vi "ATI InTrap-MALDI Explorer.vi"() -> ()   [LabVIEW 2018]
uses:
  PublicSubVI/Class/FileManager/FM/ctl/_PC_Pub_FM ctrlFileRefnumEnum.ctl
  PublicSubVI/Ctl/RegistyFunc.ctl
  PublicSubVI/Class/FileManager/FM/ctl/_PC_Pub_FM stateMachineEnum.ctl
  PublicSubVI/Class/QMH/QMH.lvclass
  PublicSubVI/Class/DataXML/DataXML.lvclass
  PublicSubVI/Class/Sig2MS/Sig2MS.lvclass
  PublicSubVI/Class/FileManager/FM.lvclass
panel:
  in  "TIC_enable":bool
  in  "Sys.Settings":bool
  in  "MS.RecipeEditor":bool
  in  "MS.Laser":bool
  in  "MS.Turbo":bool
  in  "MS.IonSource":bool
  in  "MS.Pause":bool
  in  "RemainingLoops":i32=-1
  in  "MS.Start":bool
  in  "MS.Config":bool
  in  "warning sign":bool
  in  "eng_mode_str":string
  in  "interface type":enum16{"User", "Engineer"}(ring)
  out "Stop":bool
  in  "Add GroupName":bool
  in  "Auto Index":bool
  in  "Save Config":bool
  in  "Working Folder":path
  in  "MS.AVG":u8=1 min=1 step=1
  in  "MS.Loops":i32=1 min=1 step=1
  in  "Open TempFiles":bool
  in  "Group Name Selection":string(combo)
  out "Last acq. at":timestamp
  in  "File.Save it":bool
  in  "Config Tab":enum32{"D999", "Instrument"}(tab)
  in  "D999_list":i32(listbox)=-1
  out "Instrument_param_table":string[][](table)
  in  "sys_value_list":i32(listbox)=-1
  in  "D999.Config":bool
  out "timeDomainSpec":waveform(sgl)[](graph)
  in  "AVG :":string
  out "massSpec":cluster{dbl[], sgl[]}[](graph)
  out "TIC_wfm":cluster{dbl[], sgl[]}[](graph)
  out "Ionisation":waveform(sgl)[](graph)
  out "Version :":string
  out "Interrupt Signal":bool
  in  "Smooth.edit":bool
  in  "Time domain":bool
  in  "SigProc":bool
  in  "Pressure:":string
  out "# Signal in Queue":u8(slide) scale=0.0..20.0
  out "# signal in NS":u8(slide) scale=0.0..20.0
  in  "Firmware :":string="Open Variable Connection in _PC_RTLoop_ReadCurrentMSEvent.vi->ATI InTrap-MALDI Explorer.vi"
  in  "SysMsg":string="System disconnected"
  out "Network\nstream":bool
  # "TIC"
  # "System"
  # "MSScript"
  # "MS Periphery"
  # "MS Cmd"
  # "Advanced"
  # "File Mgmt."
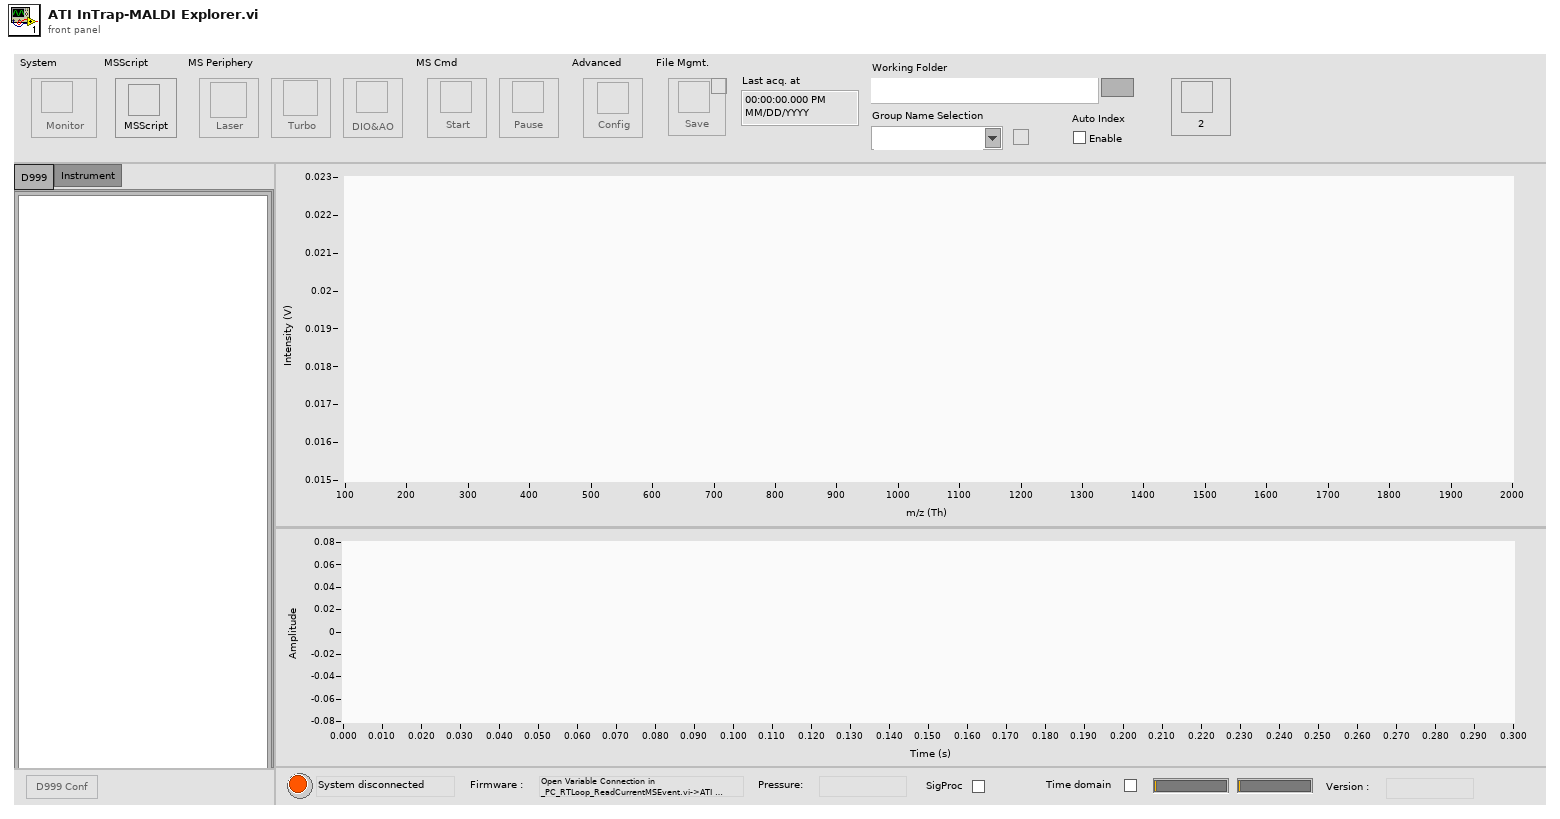
[diagram p1: front panel]
types:
  T1 = cluster{"File.Save it":refnum<vi>, "# Signal in Queue":refnum<vi>, "TIC":refnum<vi>, "Last acq. at":refnum<vi>, "sysValList":refnum<vi>, "signWarning":refnum<vi>, "MS.Pause":refnum<vi>}
  T2 = cluster{"massSpec":refnum<vi>, "timeDomainSpec":refnum<vi>, "Ionisation":refnum<vi>, "Interrupt Signal":refnum<vi>, "AVG":refnum<vi>}
  T3 = enum8{"Enabled", "Disabled", "Disabled and Grayed Out"}
  T4 = cluster{"# signal in NS":refnum<vi>, "# Signal in Queue":refnum<vi>, "MS.Start":refnum<vi>, "MS.Pause":refnum<vi>, "RemainingLoops":refnum<vi>, "Group Name Selection":refnum<vi>, "Add GroupName":refnum<vi>, "Working Folder":refnum<vi>}
  T5 = cluster{"MainVI Ref":refnum<vi>, "D999_list":refnum<vi>, "instr_param_table":refnum<vi>, "sys_value_list":refnum<vi>, "Ionisation":refnum<vi>, "SigProc":refnum<vi>, "Config Tab":refnum<vi>, "MS.RecipeEditor":refnum<vi>, "Open TempFiles":refnum<vi>, "DAQ.Config":refnum<vi>, "Mass spectrum":refnum<vi>, "TIC":refnum<vi>, "fileRefnum":cluster{"folderPath":path, "dataName":string, "fileNameRefnum":refnum<vi>, "workFolderRefnum":refnum<vi>, "openTempFile":refnum<vi>}}
  T6 = cluster{"folderPath":path, "dataName":string, "fileNameRefnum":refnum<vi>, "workFolderRefnum":refnum<vi>, "openTempFile":refnum<vi>}
  T7 = enum16{"init", "loadScript", "newScript", "runScript", "close"}
  T8 = enum16{"None", "Init", "Write", "Read", "PauseRead", "FinishCheck"}
  T9 = cluster{"Method.Path":refnum<data-value>, "MS.Continue":refnum<data-value>, "MS.Loops":refnum<data-value>, "MS.AVG":refnum<data-value>}
  T10 = typedef "_PC_Pub_FM stateMachineEnum.ctl" = enum16{"none", "init", "reset_t0", "openTDMS", "writeTDMS", "closeTDMS", "readTDMS", "getDataItems"}
  T11 = typedef "_PC_Pub_FM ctrlFileRefnumEnum.ctl" = enum16{"init", "checkFileName", "updFileName", "updWorkFolder", "updDataItems", "addNewFileName", "addSerialNum"}
  T12 = typedef "RegistyFunc.ctl" = enum16{"None", "FileAutoSave", "FileNoise", "FileSN", "ExeStatu", "WorkFolderPath", "MethodPath", "AVGItem", "LoopItem", "AutoRun", "BGColor", "LineColor", "LineWidth", "XGrid", "YGrid", "DeviceRefnum"}
  T13 = cluster{"BGColor":u32, "GridX":bool, "GridY":bool, "LineColorArray":u32[], "LineWidthArray":u8[]}
  T14 = typedef "LVPoint32TypeDef.ctl" = cluster{"Horizontal":i32, "Vertical":i32}
  T15 = typedef "LVRowAndColumnTypeDef.ctl" = cluster{"Row":i32, "Column":i32}
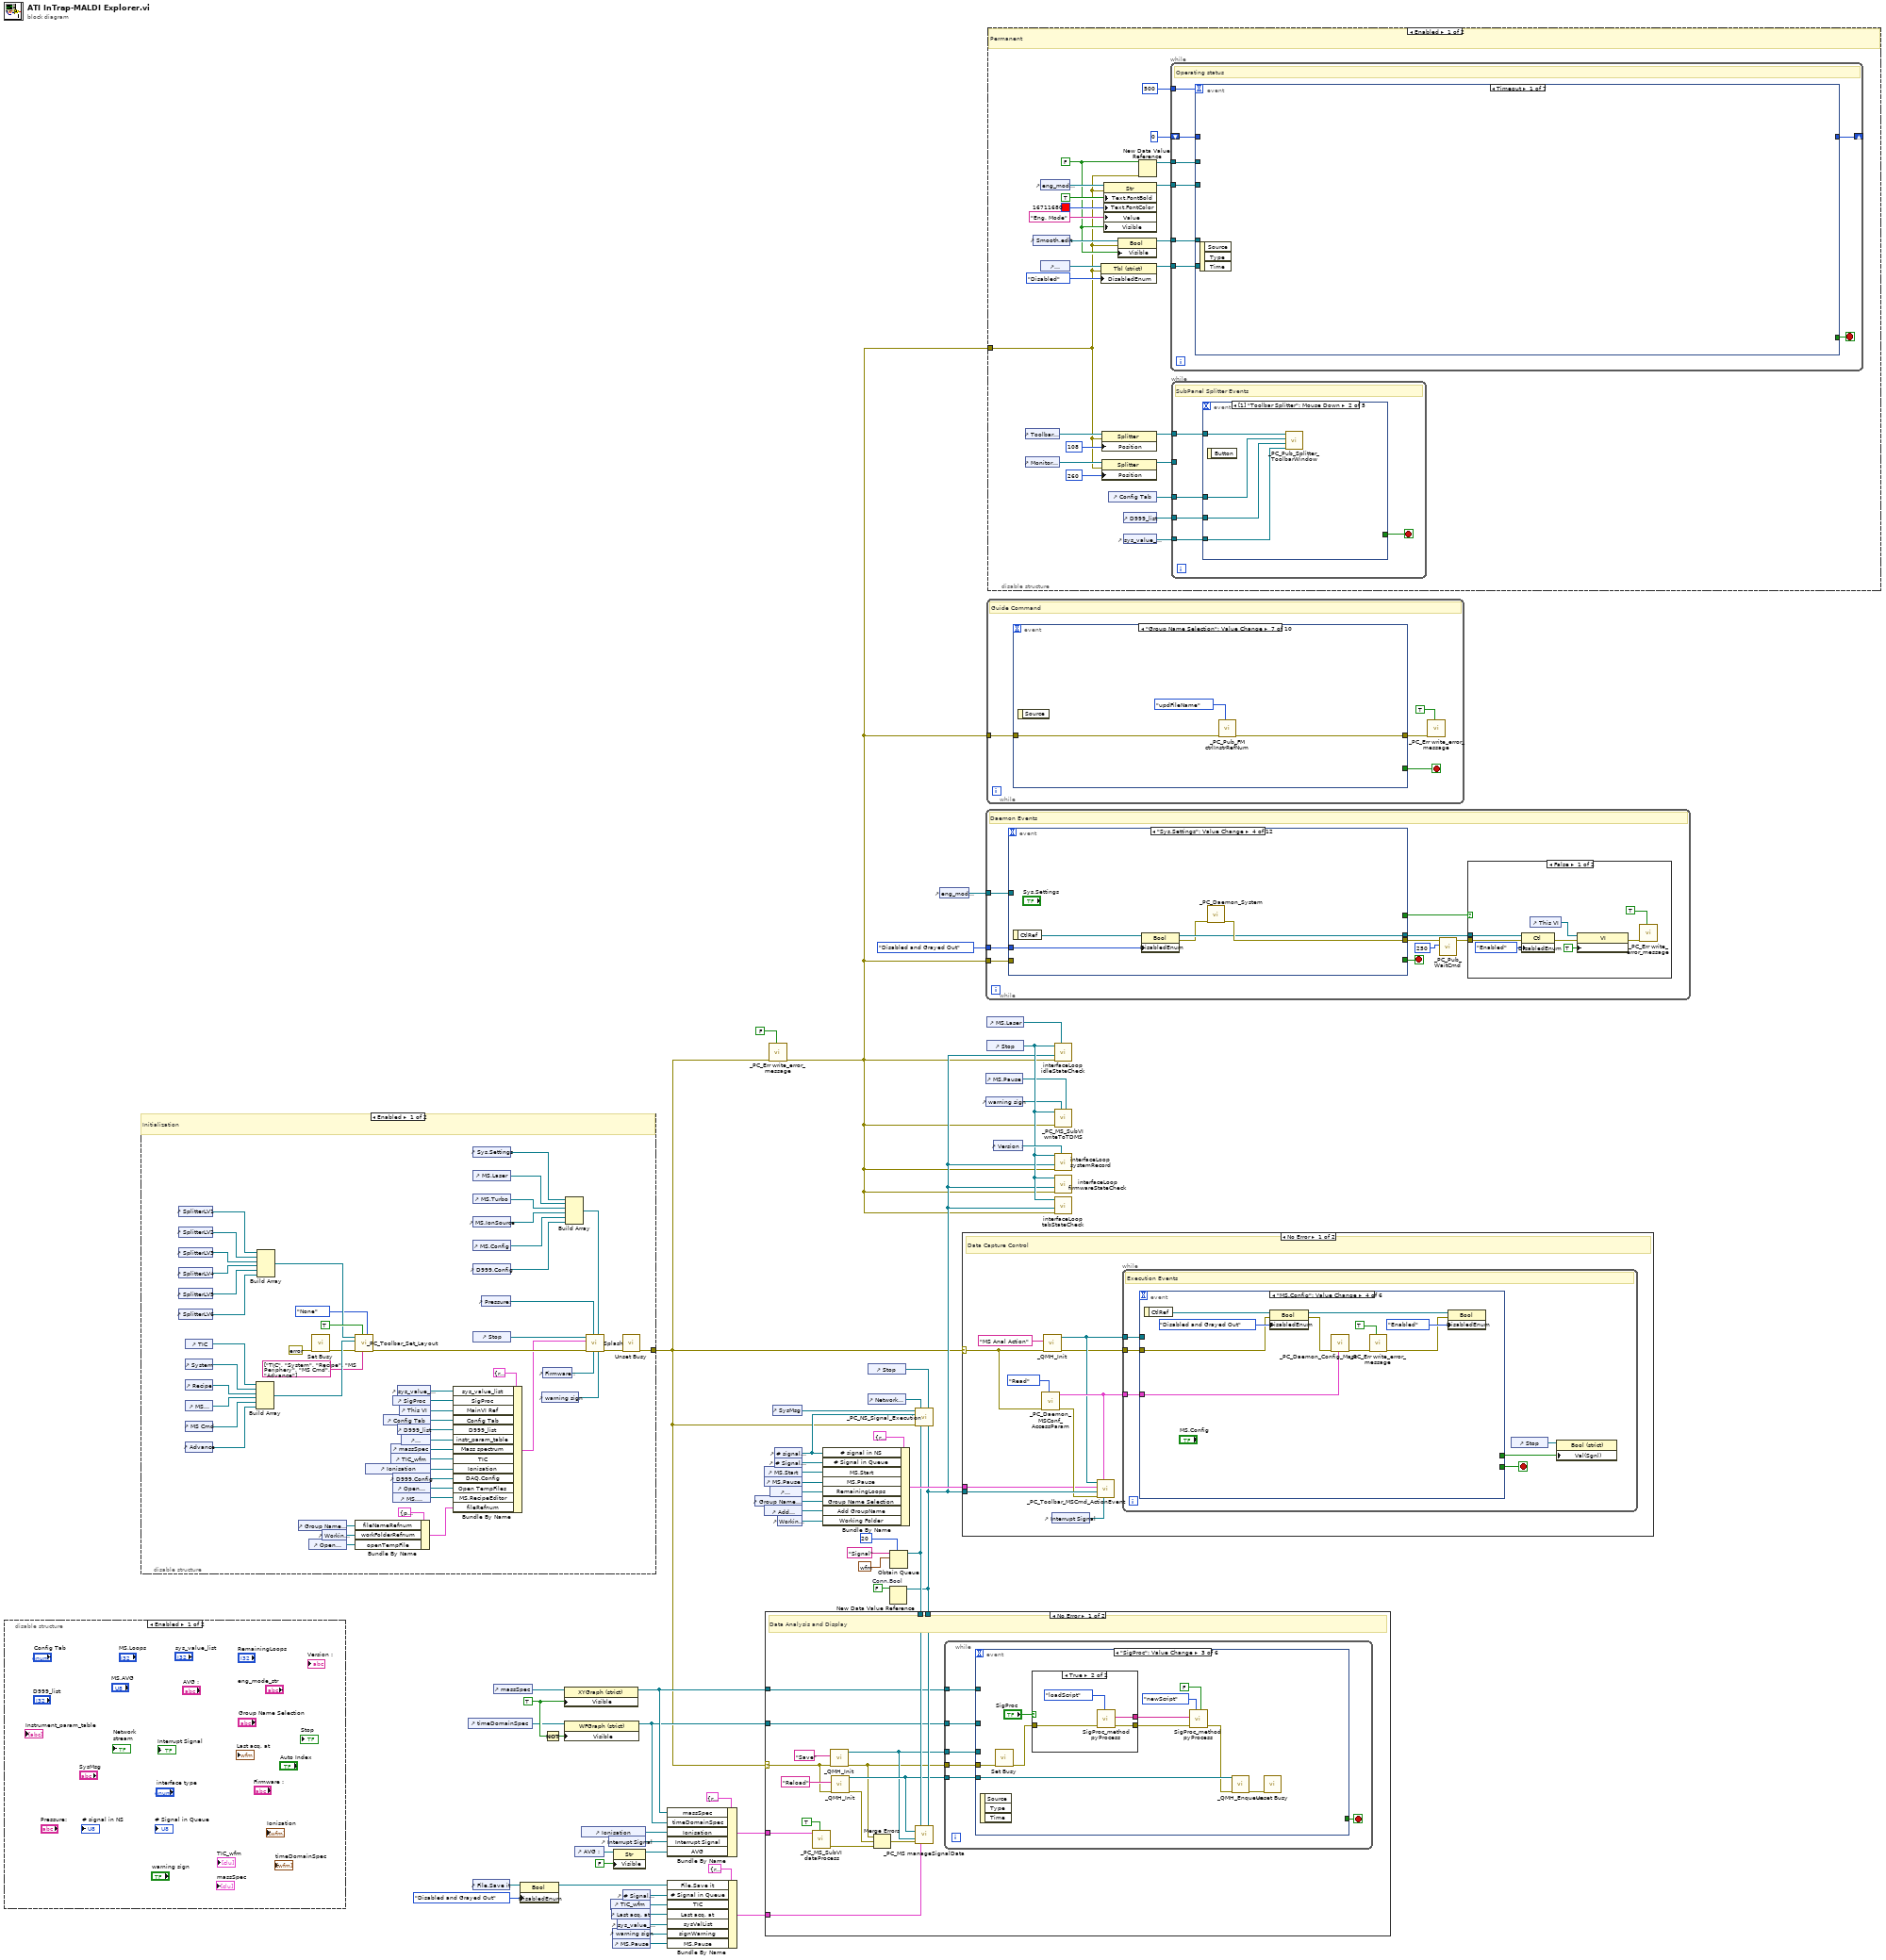
[diagram p0: block diagram]
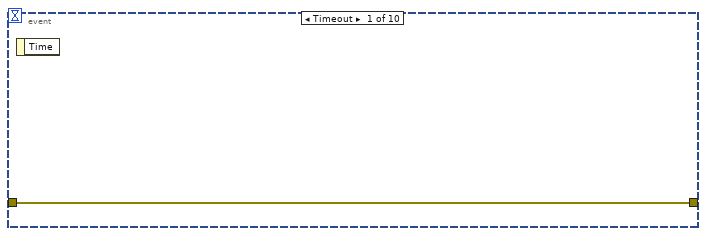
[diagram p2: hidden frame]
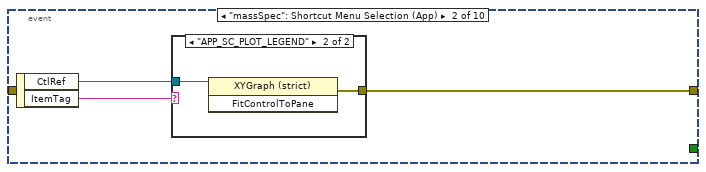
[diagram p3: hidden frame]
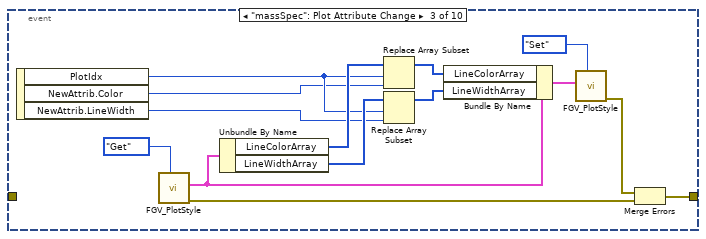
[diagram p5: hidden frame]
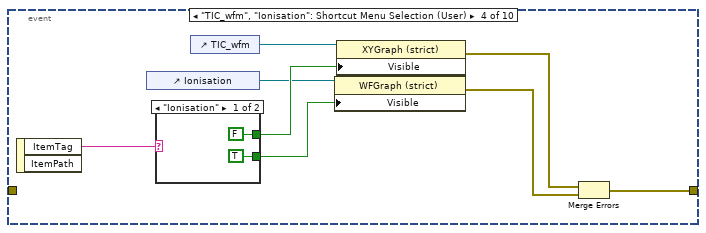
[diagram p6: hidden frame]
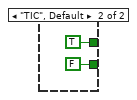
[diagram p7: hidden frame]
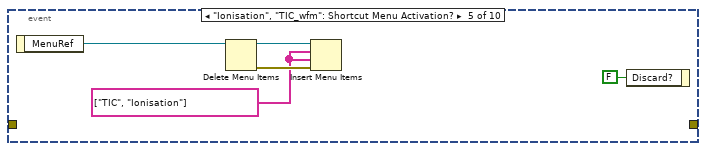
[diagram p8: hidden frame]
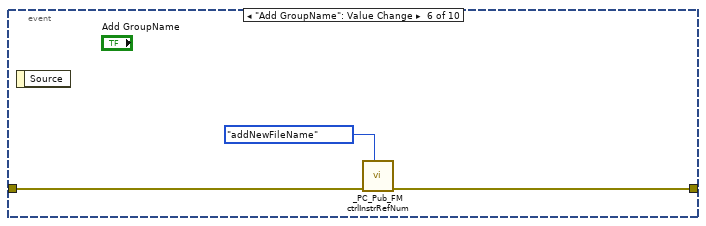
[diagram p9: hidden frame]
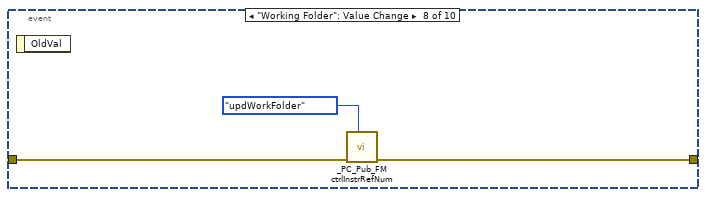
[diagram p10: hidden frame]
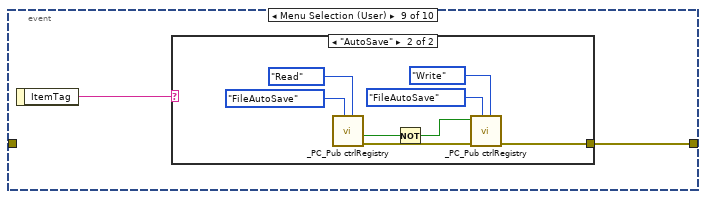
[diagram p11: hidden frame]
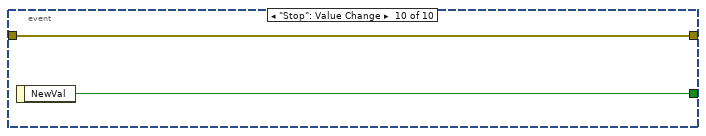
[diagram p13: hidden frame]
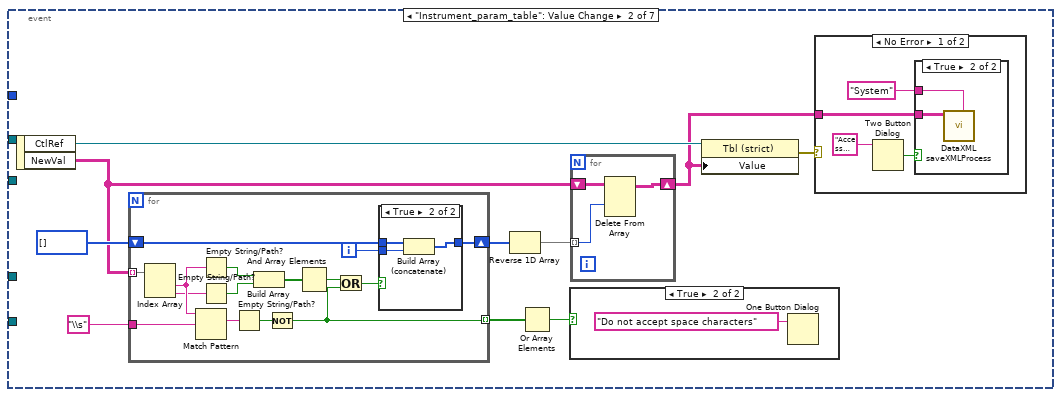
[diagram p14: hidden frame]
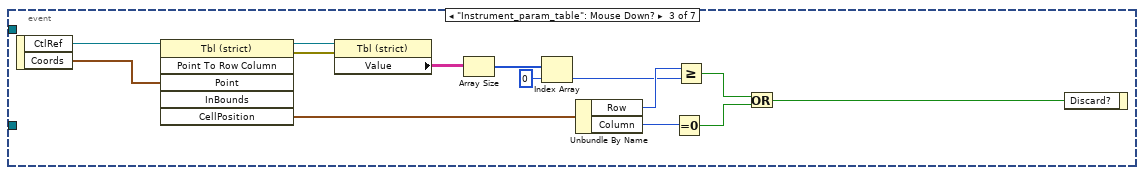
[diagram p19: hidden frame]
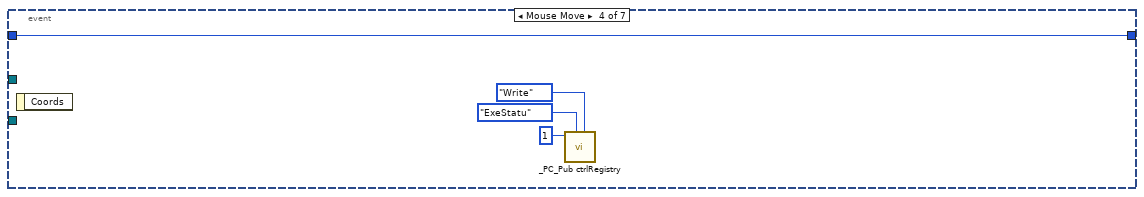
[diagram p20: hidden frame]
diagram:
  w26 = TRUE ("Visible")
  n1 = disable-structure shown="Enabled" {
    frame Enabled {
    }
    frame Disabled {
    }
  }
  n2 = disable-structure shown="Enabled" {
    disable-tunnel: [w105 _] -> w2
    frame Enabled {
      # "Initialization"
      n3 = control-ref of="SplitterLV1"() -> (w99:refnum<vi>)
      n4 = control-ref of="SplitterLV2"() -> (w98:refnum<vi>)
      n5 = control-ref of="SplitterLV3"() -> (w97:refnum<vi>)
      n6 = control-ref of="SplitterLV4"() -> (w96:refnum<vi>)
      n7 = control-ref of="SplitterLV5"() -> (w95:refnum<vi>)
      n8 = control-ref of="SplitterLV6"() -> (w94:refnum<vi>)
      n9 = control-ref of="TIC"() -> (w93:refnum<vi>)
      n10 = control-ref of="System"() -> (w92:refnum<vi>)
      n11 = control-ref of="Recipe"() -> (w91:refnum<vi>)
      n12 = control-ref of="MS Periphery"() -> (w90:refnum<vi>)
      n13 = control-ref of="MS Cmd"() -> (w88:refnum<vi>)
      n14 = control-ref of="Advance"() -> (w89:refnum<vi>)
      n15 = Build Array(w93, w92, w91, w90, w88, w89) -> (w86:refnum<vi>[])
      n16 = Build Array(w99, w98, w97, w96, w95, w94) -> (w84:refnum<vi>[])
      n17 = control-ref of="Group Name Selection"() -> (w82:refnum<vi>)
      n18 = control-ref of="Open TempFiles"() -> (w57:refnum<vi>)
      n19 = call <vilib>:"Set Busy.vi"("error in (no error)"=errorcluster {"status"=FALSE, "code"=0, "source"=""}) -> ("error out"=w81:errorcluster)  [unwired: 9 in, 1 out]
      n20 = control-ref of="Working Folder"() -> (w58:refnum<vi>)
      n21 = call "_PC_Toolbar_Set_Layout.vi"("MachineType"=enum16{"None", "MALDI", "ESI"}."None", "TagArray"=string[] ["TIC", "System", "Recipe", "MS Periphery", "MS Cmd", "Advance"], "Init?(F)"=TRUE, "error in (no error)"=w81, "PanelRef_Array"=w86, "SplitterRef_Array"=w84) -> ("error out"=w69:errorcluster)  [unwired: 5 in]
      n22 = Bundle By Name(cluster=T6 {"folderPath"=path "", "dataName"="", "fileNameRefnum"=refnum, "workFolderRefnum"=refnum, "openTempFile"=refnum} ("fileRefnum"), "fileNameRefnum"=w82, "workFolderRefnum"=w58, "openTempFile"=w57) -> (w56:T6)
      n23 = control-ref of="Ionisation"() -> (w100:refnum<vi>)
      n24 = control-ref of="Config Tab"() -> (w67:refnum<vi>)
      n25 = control-ref of="massSpec"() -> (w102:refnum<vi>)
      n26 = control-ref of="TIC_wfm"() -> (w101:refnum<vi>)
      n27 = control-ref of="SigProc"() -> (w64:refnum<vi>)
      n28 = control-ref of="D999.Config"() -> (w80:refnum<vi>)
      n29 = control-ref of="Open TempFiles"() -> (w79:refnum<vi>)
      n30 = control-ref of="MS.RecipeEditor"() -> (w78:refnum<vi>)
      n31 = control-ref of="sys_value_list"() -> (w63:refnum<vi>)
      n32 = control-ref of="D999_list"() -> (w103:refnum<vi>)
      n33 = control-ref of="This VI"() -> (w77:refnum<vi>)
      n34 = control-ref of="Instrument_param_table"() -> (w65:refnum<vi>)
      n35 = Bundle By Name(cluster=T5 {"MainVI Ref"=refnum, "D999_list"=refnum, "instr_param_table"=refnum, "sys_value_list"=refnum, "Ionisation"=refnum, "SigProc"=refnum, "Config Tab"=refnum, "MS.RecipeEditor"=refnum, "Open TempFiles"=refnum, "DAQ.Config"=refnum, "Mass spectrum"=refnum, "TIC"=refnum, "fileRefnum"={"folderPath"=path "", "dataName"="", "fileNameRefnum"=refnum, "workFolderRefnum"=refnum, "openTempFile"=refnum}} ("Init Ref"), "sys_value_list"=w63, "SigProc"=w64, "MainVI Ref"=w77, "Config Tab"=w67, "D999_list"=w103, "instr_param_table"=w65, "Mass spectrum"=w102, "TIC"=w101, "Ionisation"=w100, "DAQ.Config"=w80, "Open TempFiles"=w79, "MS.RecipeEditor"=w78, "fileRefnum"=w56) -> (w55:T5)
      n36 = control-ref of="Sys.Settings"() -> (w75:refnum<vi>)
      n37 = control-ref of="MS.Laser"() -> (w74:refnum<vi>)
      n38 = control-ref of="MS.Turbo"() -> (w73:refnum<vi>)
      n39 = control-ref of="MS.IonSource"() -> (w72:refnum<vi>)
      n40 = control-ref of="MS.Config"() -> (w66:refnum<vi>)
      n41 = control-ref of="D999.Config"() -> (w71:refnum<vi>)
      n42 = control-ref of="Stop"() -> (w68:refnum<vi>)
      n43 = control-ref of="Pressure:"() -> (w70:refnum<vi>)
      n44 = control-ref of="warning sign"() -> (w61:refnum<vi>)
      n45 = control-ref of="Firmware :"() -> (w62:refnum<vi>)
      n46 = Build Array(w75, w74, w73, w72, w66, w71) -> (w104:refnum<vi>[])
      n47 = call "Splash.vi"("warning sign"=w61, "Cluster control array"=w104, "Firmware :"=w62, "Pressure:"=w70, "error in (no error)"=w69, "Init Ref"=w55, "Stop"=w68) -> ("error out"=w60:errorcluster)  [unwired: 4 in]
      n48 = call <vilib>:"Unset Busy.vi"("error in (no error)"=w60) -> ("error out"=w105:errorcluster)  [unwired: 10 in]
    }
    frame Disabled {
    }
  }
  n49 = control-ref of="timeDomainSpec"() -> (w23:refnum<vi>)
  n50 = control-ref of="File.Save it"() -> (w49:refnum<vi>)
  n51 = control-ref of="massSpec"() -> (w24:refnum<vi>)
  n52 = property class="Bool"(reference=w49, "DisabledEnum"=T3."Disabled and Grayed Out" ("Disabled")) -> (reference out=w48:refnum<vi>)  [unwired: 1 in, 1 out]
  n53 = Not(x=w26) -> (.not. x?=w25:bool)
  n54 = property class="XYGraph (strict)"(reference=w24, "Visible"=w26) -> (reference out=w22:refnum<vi>)  [unwired: 1 in, 1 out]
  n55 = property class="WFGraph (strict)"(reference=w23, "Visible"=w25) -> (reference out=w19:refnum<vi>)  [unwired: 1 in, 1 out]
  n56 = control-ref of="AVG :"() -> (w20:refnum<vi>)
  n57 = control-ref of="Ionisation"() -> (w21:refnum<vi>)
  n58 = control-ref of="Interrupt Signal"() -> (w17:refnum<vi>)
  n59 = control-ref of="TIC_wfm"() -> (w51:refnum<vi>)
  n60 = control-ref of="Last acq. at"() -> (w53:refnum<vi>)
  n61 = control-ref of="warning sign"() -> (w14:refnum<vi>)
  n62 = control-ref of="MS.Pause"() -> (w13:refnum<vi>)
  n63 = property class="Str"(reference=w20, "Visible"=FALSE) -> (reference out=w16:refnum<vi>)  [unwired: 1 in, 1 out]
  n64 = control-ref of="sys_value_list"() -> (w15:refnum<vi>)
  n65 = control-ref of="# Signal in Queue"() -> (w52:refnum<vi>)
  n66 = Bundle By Name(cluster=T1 {"File.Save it"=refnum, "# Signal in Queue"=refnum, "TIC"=refnum, "Last acq. at"=refnum, "sysValList"=refnum, "signWarning"=refnum, "MS.Pause"=refnum}, "File.Save it"=w48, "# Signal in Queue"=w52, "TIC"=w51, "Last acq. at"=w53, "sysValList"=w15, "signWarning"=w14, "MS.Pause"=w13) -> (w42:T1)
  n67 = Bundle By Name(cluster=T2 {"massSpec"=refnum, "timeDomainSpec"=refnum, "Ionisation"=refnum, "Interrupt Signal"=refnum, "AVG"=refnum} ("Reference"), "massSpec"=w22, "timeDomainSpec"=w19, "Ionisation"=w21, "Interrupt Signal"=w17, "AVG"=w16) -> (w40:T2)
  n68 = control-ref of="Group Name Selection"() -> (w6:refnum<vi>)
  n69 = control-ref of="MS.Start"() -> (w31:refnum<vi>)
  n70 = control-ref of="MS.Pause"() -> (w27:refnum<vi>)
  n71 = control-ref of="Add GroupName"() -> (w5:refnum<vi>)
  n72 = call "_PC_Err write_error_message.vi"("show msg( T )"=FALSE, "error in"=w2) -> ("error out"=w1:errorcluster)  [unwired: 9 in]
  n73 = control-ref of="RemainingLoops"() -> (w33:refnum<vi>)
  n74 = control-ref of="SysMsg"() -> (w44:refnum<vi>)
  n75 = control-ref of="# signal in NS"() -> (w43:refnum<vi>)
  n76 = control-ref of="# Signal in Queue"() -> (w46:refnum<vi>)
  n77 = control-ref of="Working Folder"() -> (w4:refnum<vi>)
  n78 = Bundle By Name(cluster=T4 {"# signal in NS"=refnum, "# Signal in Queue"=refnum, "MS.Start"=refnum, "MS.Pause"=refnum, "RemainingLoops"=refnum, "Group Name Selection"=refnum, "Add GroupName"=refnum, "Working Folder"=refnum} ("Cluster"), "# signal in NS"=w43, "# Signal in Queue"=w46, "MS.Start"=w31, "MS.Pause"=w27, "RemainingLoops"=w33, "Group Name Selection"=w6, "Add GroupName"=w5, "Working Folder"=w4) -> (w45:T4)
  n79 = control-ref of="Stop"() -> (w32:refnum<vi>)
  n80 = control-ref of="Network\nstream"() -> (w47:refnum<vi>)
  n81 = New Data Value Reference "Conn.Bool"(data value=FALSE) -> (data value reference=w9:refnum<data-value>)  [unwired: 1 in, 1 out]
  n82 = Obtain Queue(max queue size (-1, unlimited)=20, name (unnamed)="Signal", element data type=waveform(sgl) {"t0"=timestamp(0 s since 1904-01-01), "dt"=1.0, "Y"=[]} ("element")) -> (queue out=w35:refnum<queue>)  [unwired: 2 in, 2 out]
  n83 = case shown="No Error" w2 {
    selector: w2 -> [w116 _]
    tunnel: w35 -> [w121 _]
    tunnel: w9 -> [w120 _]
    tunnel: w42 -> [w115 _]
    tunnel: w40 -> [w113 _]
    tunnel: w22 -> [w108 _]
    tunnel: w19 -> [w107 _]
    frame No Error {
      # "Data Analysis and Display"
      n84 = call "_PC_MS_SubVI dataProcess.vi"("Init?(F)"=TRUE, "Reference"=w113) -> ("error out"=w110:errorcluster)  [unwired: 8 in, 1 out]
      n85 = call "_QMH_Init.vi"("error in (no error)"=w116, "name (unnamed)"="Save") -> ("error out"=w112:errorcluster, "QMH out"=w114:refnum<class "QMH.lvclass">)  [unwired: 8 in]
      n86 = call "_QMH_Init.vi"("error in (no error)"=w116, "name (unnamed)"="Reload") -> ("error out"=w111:errorcluster, "QMH out"=w117:refnum<class "QMH.lvclass">)  [unwired: 8 in]
      n87 = Merge Errors(w112, w111, w110) -> (w109:errorcluster)
      n88 = call "_PC_MS manageSignalData.vi"("Sig Queue"=w121, "Conn_Bool"=w120, "Reload_QMH"=w117, "Save_QMH"=w114, "error in (no error)"=w109, "exeObjRefnum"=w115) -> ()  [unwired: 10 in]
      n89 = while {
        tunnel: w117 -> [w127]
        tunnel: w114 -> [w126]
        tunnel: w112 -> [w125]
        tunnel: w108 -> [w123]
        tunnel: w107 -> [w122]
        stop <- w124 stop-if-true
        n90 = event shown="[2] \"SigProc\": Value Change" {
          selector: _ -> [_ _ _ _ _ _]
          dyn-events: _ -> [_ _ _ _ _ _]
          timeout: _ -> [_ _ _ _ _ _]
          tunnel: w127 -> [_ w135 w147 _ w162 _]
          tunnel: w126 -> [_ _ _ w158 _ _]
          tunnel: w125 -> [_ _ w145 w157 w161 _]
          tunnel: [_ _ _ _ _ w163] -> w124
          tunnel: w123 -> [_ w134 _ _ _ _]
          tunnel: w122 -> [_ w133 _ _ _ _]
          event Timeout {
            n91 = event-data() -> ()  [unwired: 1 in, 3 out]
          }
          event "Time domain": Value Change {
            n92 = event-data() -> ()  [unwired: 1 in, 3 out]
            n93 = Not(x="Time domain") -> (.not. x?=w132:bool)
            n94 = property class="WFGraph (strict)"(reference=w133, "Visible"="Time domain") -> (reference out=w129:refnum<vi>)  [unwired: 1 in, 1 out]
            n95 = property class="XYGraph (strict)"(reference=w134, "Visible"=w132) -> (reference out=w130:refnum<vi>)  [unwired: 1 in, 1 out]
            n96 = case shown="False" "Time domain" {
              tunnel: w130 -> [w138 _]
              tunnel: w129 -> [_ w141]
              tunnel: [w136 w139] -> w128
              frame False {
                n97 = property class="XYGraph (strict)"(reference=w138, "Value"=cluster{dbl[], sgl[]}[] []) -> (error out=w136:errorcluster)  [unwired: 1 in, 1 out]
              }
              frame True {
                n98 = property class="WFGraph (strict)"(reference=w141, "Value"=waveform(dbl)[] []) -> (error out=w139:errorcluster)  [unwired: 1 in, 1 out]
              }
            }
            n99 = call "_QMH_Enqueue.vi"("error in (no error)"=w128, "QMH in"=w135) -> ()  [unwired: 8 in, 2 out]
          }
          event "SigProc": Value Change {
            n100 = event-data() -> ()  [unwired: 1 in, 3 out]
            n101 = call <vilib>:"Set Busy.vi"("error in (no error)"=w145) -> ("error out"=w144:errorcluster)  [unwired: 9 in, 1 out]
            n102 = case shown="True" "SigProc" {
              tunnel: [_ w155] -> w149
              tunnel: [w152 w154] -> w148
              tunnel: w144 -> [w152 w153]
              frame False {
              }
              frame True {
                n103 = call "SigProc_method pyProcess.vi"("func"=T7."loadScript", "error in (no error)"=w153) -> ("error out"=w154:errorcluster, "pyCode"=w155:string)  [unwired: 6 in, 2 out]
              }
            }
            n104 = call "SigProc_method pyProcess.vi"("replace?(T)"=FALSE, "func"=T7."newScript", "error in (no error)"=w148, "newScriptCode"=w149) -> ("error out"=w146:errorcluster)  [unwired: 4 in, 3 out]
            n105 = call "_QMH_Enqueue.vi"("error in (no error)"=w146, "QMH in"=w147) -> ("error out"=w143:errorcluster)  [unwired: 8 in, 1 out]
            n106 = call <vilib>:"Unset Busy.vi"("error in (no error)"=w143) -> ()  [unwired: 10 in, 1 out]
          }
          event "File.Save it": Value Change {
            n107 = event-data() -> ()  [unwired: 1 in, 1 out]
            n108 = call "_QMH_Enqueue.vi"("error in (no error)"=w157, "Msg"="Save", "QMH in"=w158) -> ()  [unwired: 7 in, 2 out]
          }
          event "Smooth.edit": Value Change {
            n109 = event-data() -> ()  [unwired: 1 in, 1 out]
            n110 = call "Sig2MS dialogPyScript.vi"("error in (no error)"=w161) -> ("error out"=w160:errorcluster)  [unwired: 10 in]
            n111 = call "_QMH_Enqueue.vi"("error in (no error)"=w160, "QMH in"=w162) -> ()  [unwired: 8 in, 2 out]
          }
          event "Stop": Value Change {
            n112 = event-data() -> ("NewVal"=w163:bool)  [unwired: 1 in]
          }
        }
      }
    }
    frame Error {
    }
  }
  n113 = call "_PC_NS_Signal_Execution.vi"("SysMsg"=w44, "Network\nstream"=w47, "Stop"=w32, "# signal in NS"=w43, "error in (no error)"=w2, "Sig Queue"=w35, "Conn_Bool"=w9) -> ()  [unwired: 9 in]
  n114 = control-ref of="eng_mode_str"() -> (w30:refnum<vi>)
  n115 = case shown="No Error" w2 {
    selector: w2 -> [w166 w240]
    tunnel: w9 -> [w172 _]
    tunnel: w45 -> [w164 _]
    frame No Error {
      # "Data Capture Control"
      n116 = call "_PC_Daemon_MSConf_AccessParam.vi"("Function"=enum16{"Write", "Read"}."Read", "error in (no error)"=w166) -> ("error out"=w168:errorcluster, "exe param memory"=w169:T9)  [unwired: 8 in]
      n117 = call "_QMH_Init.vi"("error in (no error)"=w166, "name (unnamed)"="MS Anal Action") -> ("error out"=w165:errorcluster, "QMH out"=w167:refnum<class "QMH.lvclass">)  [unwired: 8 in]
      n118 = control-ref of="Interrupt Signal"() -> (w171:refnum<vi>)
      n119 = call "_PC_Toolbar_MSCmd_ActionEvent.vi"("Interrupt Signal"=w171, "exe param memory"=w169, "error in (no error)"=w168, "Conn_Bool"=w172, "Cluster"=w164, "QMH In"=w167) -> ()  [unwired: 6 in]
      n120 = while {
        tunnel: w167 -> [w179]
        tunnel: w165 -> [w178]
        tunnel: w169 -> [w177]
        stop <- w174 stop-if-true
        # "Execution Events"
        n121 = event shown="[3] \"MS.Config\": Value Change" {
          selector: _ -> [_ _ _ _ _ _]
          dyn-events: _ -> [_ _ _ _ _ _]
          timeout: _ -> [_ _ _ _ _ _]
          tunnel: w179 -> [_ w195 w209 _ w222 _]
          tunnel: w178 -> [_ w189 w206 w215 w221 _]
          tunnel: w177 -> [_ w192 _ w220 w225 _]
          tunnel: [_ _ _ _ _ TRUE ("stop")] -> w174
          tunnel: [_ _ _ _ TRUE _] -> w175
          event Timeout {
            n122 = event-data() -> ()  [unwired: 1 in, 1 out]
          }
          event "MS.Start": Value Change {
            n123 = event-data() -> ()  [unwired: 1 in, 1 out]
            n124 = Unbundle By Name(w192) -> ("MS.Continue"=w191:refnum<data-value>)
            n125 = call <vilib>:"Set Busy.vi"("error in (no error)"=w189) -> ("error out"=w188:errorcluster)  [unwired: 9 in, 1 out]
            n126 = control-ref of="Ionisation"() -> (w183:refnum<vi>)
            n127 = in-place {
              in-place-border: [w204] -> w199
              in-place-border: w188 -> [_]
              n128 = in-place-dvr #1(w191) -> (w204:bool)  [unwired: 1 out]
              n129 = in-place-dvr #1(w204) -> (w190:errorcluster)  [unwired: 1 out]
            }
            n130 = control-ref of="massSpec"() -> (w194:refnum<vi>)
            n131 = control-ref of="TIC_wfm"() -> (w193:refnum<vi>)
            n132 = control-ref of="Auto Index"() -> (w184:refnum<vi>)
            n133 = Select(t="StartInf" ("Msg"), s=w199, f="Start" ("Msg")) -> (s? t:f=w196:string)
            n134 = call "_PC_MS_SubVI exeInit.vi"("Auto Index"=w184, "error in (no error)"=w190, "Ionisation Ref"=w183, "TIC Ref"=w193, "Mass Spetrum Ref"=w194) -> ("error out"=w182:errorcluster)  [unwired: 6 in]
            n135 = case shown="No Error" w182 {
              selector: w182 -> [w201 _]
              tunnel: w196 -> [w203 _]
              tunnel: w195 -> [w202 _]
              tunnel: [w200 _] -> w187
              frame No Error {
                n136 = call "_QMH_Enqueue.vi"("error in (no error)"=w201, "Msg"=w203, "QMH in"=w202) -> ("error out"=w200:errorcluster)  [unwired: 7 in, 1 out]
              }
              frame Error {
              }
            }
            n137 = call <vilib>:"Clear Errors.vi"("error in (no error)"=w182) -> ("error out"=w181:errorcluster)  [unwired: 5 in, 1 out]
            n138 = call "_PC_Pub_FM ctrlTempStateMachine.vi"("function"=T8."Init", "error in (no error)"=w181) -> ()  [unwired: 7 in, 3 out]
            n139 = call "_PC_Pub_WaitCmd.vi"("milliseconds to wait"=u32 200, "error in (no error)"=w187) -> ("error out"=w186:errorcluster)  [unwired: 9 in]
            n140 = call <vilib>:"Unset Busy.vi"("error in (no error)"=w186) -> ()  [unwired: 10 in, 1 out]
          }
          event "MS.Pause": Value Change {
            n141 = event-data() -> ("CtlRef"=w208:refnum<vi>)  [unwired: 1 in]
            n142 = property class="Bool (strict)"(reference=w208, error in=w206, "DisabledEnum"=T3."Disabled and Grayed Out" ("Disabled")) -> (error out=w205:errorcluster)  [unwired: 1 out]
            n143 = call "_QMH_Enqueue.vi"("error in (no error)"=w205, "Msg"="Pause", "QMH in"=w209) -> ()  [unwired: 7 in, 2 out]
          }
          event "MS.Config": Value Change {
            n144 = event-data() -> ("CtlRef"=w216:refnum<vi>)  [unwired: 1 in]
            n145 = property class="Bool"(reference=w216, error in=w215, "DisabledEnum"=T3."Disabled and Grayed Out" ("Disabled")) -> (reference out=w213:refnum<vi>, error out=w214:errorcluster)
            n146 = call "_PC_Daemon_Config_Mass.vi"("exe param memory"=w220, "error in (no error)"=w214) -> ("error out"=w219:errorcluster)  [unwired: 9 in]
            n147 = call "_PC_Err write_error_message.vi"("show msg( T )"=TRUE, "error in"=w219) -> ("error out"=w211:errorcluster)  [unwired: 9 in]
            n148 = property class="Bool"(reference=w213, error in=w211, "DisabledEnum"=T3."Enabled" ("Disabled")) -> ()  [unwired: 2 out]
          }
          event Panel Close? {
            n149 = event-data() -> ()  [unwired: 1 in, 1 out]
            n150 = Unbundle By Name(w225) -> ("Method.Path"=w231:refnum<data-value>, "MS.Continue"=w228:refnum<data-value>, "MS.Loops"=w229:refnum<data-value>, "MS.AVG"=w230:refnum<data-value>)
            n151 = Delete Data Value Reference(data value reference=w230) -> (error out=w232:errorcluster)  [unwired: 1 in, 1 out]
            n152 = Delete Data Value Reference(data value reference=w229, error in=w232) -> (error out=w233:errorcluster)  [unwired: 1 out]
            n153 = Delete Data Value Reference(data value reference=w228, error in=w233) -> (error out=w234:errorcluster)  [unwired: 1 out]
            n154 = call "_QMH_Enqueue.vi"("error in (no error)"=w221, "Msg"="Close", "QMH in"=w222) -> ("error out"=w235:errorcluster)  [unwired: 7 in, 1 out]
            n155 = Delete Data Value Reference(data value reference=w231, error in=w234) -> (error out=w236:errorcluster)  [unwired: 1 out]
            n156 = Merge Errors(w235, w236) -> (w223:errorcluster)
            n157 = call "_PC_Err write_error_message.vi"("show msg( T )"=FALSE, "error in"=w223) -> ()  [unwired: 9 in, 1 out]
            n158 = event-data() -> ()  [unwired: 2 in, 1 out]
          }
          event Panel Close {
            n159 = event-data() -> ()  [unwired: 1 in, 1 out]
          }
        }
        n160 = control-ref of="Stop"() -> (w176:refnum<vi>)
        n161 = property class="Bool (strict)"(reference=w176, "Val(Sgnl)"=w175) -> ()  [unwired: 1 in, 2 out]
      }
    }
    frame Error {
      n162 = call "_PC_Err write_error_message.vi"("show msg( T )"=FALSE, "error in"=w240) -> ("error out"=w238:errorcluster)  [unwired: 9 in]
      n163 = flat-sequence {
        tunnel: w238 -> [_]
        frame #0 {
          n164 = control-ref of="This VI"() -> (w241:refnum<vi>)
          n165 = invoke class="VI" method="FP.Close"(reference=w241) -> ()  [unwired: 2 in, 3 out]
        }
      }
    }
  }
  n166 = while {
    tunnel: w1 -> [w243]
    tunnel: w30 -> [w244]
    tunnel: T3."Disabled and Grayed Out" ("Disabled") -> [w242]
    stop <- w249 stop-if-true
    # "Daemon Events"
    n167 = event shown="[3] \"Sys.Settings\": Value Change" {
      selector: _ -> [_ _ _ _ _ _ _ _ _ _ _ _]
      dyn-events: _ -> [_ _ _ _ _ _ _ _ _ _ _ _]
      timeout: _ -> [_ _ _ _ _ _ _ _ _ _ _ _]
      tunnel: [_ w260 w266 w272 w280 w283 w289 w297 w300 w306 w330 _] -> w250
      tunnel: [_ w263 w270 w275 w277 w287 w293 w299 w304 w310 w317 _] -> w245
      tunnel: [_ _ _ _ _ _ _ _ _ _ _ w334] -> w249
      tunnel: [_ _ _ _ _ _ _ _ _ _ _ TRUE ("NewVal")] -> w246
      tunnel: w244 -> [_ _ _ _ w276 w288 w294 _ w305 _ _ _]
      tunnel: w243 -> [_ _ _ _ _ _ _ _ _ _ _ _]
      tunnel: w242 -> [_ w261 w268 w273 w281 w285 w291 w296 w302 w308 w331 _]
      event Timeout {
        n168 = event-data() -> ()  [unwired: 1 in, 1 out]
      }
      event "TIC_enable": Value Change {
        n169 = event-data() -> ("CtlRef"=w262:refnum<vi>)  [unwired: 1 in]
        n170 = property class="Bool"(reference=w262, "DisabledEnum"=w261) -> (reference out=w260:refnum<vi>, error out=w259:errorcluster)  [unwired: 1 in]
        n171 = disable-structure shown="Disabled" {
          disable-tunnel: [w265 _] -> w263
          disable-tunnel: w259 -> [w264 _]
          frame Disabled {
            n172 = call "_PC_Daemon_Chromatogram.vi"(8:w264) -> ("error out"=w265:errorcluster)  [unwired: 10 in]
          }
          frame Enabled {
          }
        }
      }
      event "Save Config": Value Change {
        n173 = event-data() -> ("CtlRef"=w269:refnum<vi>)  [unwired: 1 in]
        n174 = property class="Bool"(reference=w269, "DisabledEnum"=w268) -> (reference out=w266:refnum<vi>, error out=w267:errorcluster)  [unwired: 1 in]
        n175 = call "_PC_Daemon_Config_SaveData.vi"("error in (no error)"=w267) -> ("error out"=w270:errorcluster)  [unwired: 10 in]
      }
      event "Sys.Settings": Value Change {
        n176 = event-data() -> ("CtlRef"=w274:refnum<vi>)  [unwired: 1 in]
        n177 = property class="Bool"(reference=w274, "DisabledEnum"=w273) -> (reference out=w272:refnum<vi>, error out=w271:errorcluster)  [unwired: 1 in]
        n178 = call "_PC_Daemon_System.vi"("error in (no error)"=w271) -> ("error out"=w275:errorcluster)  [unwired: 9 in, 1 out]
      }
      event "MS.RecipeEditor": Value Change {
        n179 = event-data() -> ("CtlRef"=w282:refnum<vi>)  [unwired: 1 in]
        n180 = property class="Bool"(reference=w282, "DisabledEnum"=w281) -> (reference out=w280:refnum<vi>, error out=w278:errorcluster)  [unwired: 1 in]
        n181 = control-ref of="Network\nstream"() -> (w279:refnum<vi>)
        n182 = call "_PC_Daemon_RecipeEditor.vi"("eng_mode_str"=w276, "error in (no error)"=w278, "Network\nstream"=w279) -> ("error out"=w277:errorcluster)  [unwired: 8 in]
      }
      event "MS.Laser": Value Change {
        n183 = event-data() -> ("CtlRef"=w286:refnum<vi>)  [unwired: 1 in]
        n184 = property class="Bool"(reference=w286, "DisabledEnum"=w285) -> (reference out=w283:refnum<vi>, error out=w284:errorcluster)  [unwired: 1 in]
        n185 = call "_PC_Daemon_Laser.vi"("eng_mode_str"=w288, "error in (no error)"=w284) -> ("error out"=w287:errorcluster)  [unwired: 9 in]
      }
      event "MS.Turbo": Value Change {
        n186 = event-data() -> ("CtlRef"=w292:refnum<vi>)  [unwired: 1 in]
        n187 = property class="Bool"(reference=w292, "DisabledEnum"=w291) -> (reference out=w289:refnum<vi>, error out=w290:errorcluster)  [unwired: 1 in]
        n188 = call "_PC_Daemon_TurboPump.vi"("engModeStr"=w294, "error in (no error)"=w290) -> ("error out"=w293:errorcluster)  [unwired: 9 in]
      }
      event "D999.Config": Value Change {
        n189 = event-data() -> ("CtlRef"=w298:refnum<vi>)  [unwired: 1 in]
        n190 = property class="Bool"(reference=w298, "DisabledEnum"=w296) -> (reference out=w297:refnum<vi>, error out=w295:errorcluster)  [unwired: 1 in]
        n191 = call "_PC_Daemon_Config_D999.vi"("error in (no error)"=w295) -> ("error out"=w299:errorcluster)  [unwired: 10 in]
      }
      event "MS.IonSource": Value Change {
        n192 = event-data() -> ("CtlRef"=w303:refnum<vi>)  [unwired: 1 in]
        n193 = property class="Bool"(reference=w303, "DisabledEnum"=w302) -> (reference out=w300:refnum<vi>, error out=w301:errorcluster)  [unwired: 1 in]
        n194 = call "_PC_Daemon_AO&DO.vi"("eng_mode"=w305, "error in (no error)"=w301) -> ("error out"=w304:errorcluster)  [unwired: 9 in]
      }
      event "Pressure:": Mouse Down {
        n195 = event-data() -> ("CtlRef"=w309:refnum<vi>)  [unwired: 1 in]
        n196 = property class="Str"(reference=w309, "DisabledEnum"=w308) -> (reference out=w306:refnum<vi>, error out=w307:errorcluster)  [unwired: 1 in]
        n197 = call "_PC_Daemon_Pressurevi.vi"("Function"=enum16{"Get reference", "Show graph"}."Show graph", "error in (no error)"=w307) -> ("error out"=w310:errorcluster)  [unwired: 8 in, 1 out]
      }
      event "Open TempFiles": Value Change {
        n198 = event-data() -> ("CtlRef"=w332:refnum<vi>)  [unwired: 1 in]
        n199 = property class="Bool"(reference=w332, "DisabledEnum"=w331) -> (reference out=w330:refnum<vi>, error out=w321:errorcluster)  [unwired: 1 in]
        n200 = control-ref of="SigProc"() -> (w328:refnum<vi>)
        n201 = call "_PC_Pub_FM ctrlTempStateMachine.vi"("pause? (F)"=TRUE, "function"=T8."PauseRead", "error in (no error)"=w321) -> ("error out"=w316:errorcluster)  [unwired: 6 in, 2 out]
        n202 = property class="Bool (strict)"(reference=w328) -> ("Value"=w327:bool)  [unwired: 1 in, 2 out]
        n203 = call "_PC_Pub_WaitCmd.vi"("milliseconds to wait"=u32 500, "error in (no error)"=w316) -> ("error out"=w315:errorcluster)  [unwired: 9 in]
        n204 = call "_PC_Pub_FM stateMachine.vi"("Func"=_PC_Pub_FM_stateMachineEnum."closeTDMS", "error in (no error)"=w315) -> ("error out"=w325:errorcluster, "tdmsFilePath out"=w322:path)  [unwired: 7 in, 1 out]
        n205 = call "_PC_Daemon_SaveFiles.vi"("SigProc.Enable"=w327, "error in (no error)"=w325, "Document Path"="Working Folder") -> ("error out"=w323:errorcluster)  [unwired: 8 in]
        n206 = call "_PC_Pub_FM stateMachine.vi"("Func"=_PC_Pub_FM_stateMachineEnum."openTDMS", "error in (no error)"=w323, "tdmsFilePath in"=w322) -> ("error out"=w318:errorcluster)  [unwired: 6 in, 2 out]
        n207 = call "_PC_Pub_FM ctrlTempStateMachine.vi"("pause? (F)"=FALSE, "function"=T8."PauseRead", "error in (no error)"=w318) -> ("error out"=w317:errorcluster)  [unwired: 6 in, 2 out]
      }
      event "Stop": Value Change {
        n208 = event-data() -> ("NewVal"=w334:bool)  [unwired: 1 in]
      }
    }
    n209 = call "_PC_Pub_WaitCmd.vi"("milliseconds to wait"=u32 250, "error in (no error)"=w245) -> ("error out"=w248:errorcluster)  [unwired: 9 in]
    n210 = case shown="False" w246 {
      tunnel: w250 -> [w255 _]
      tunnel: w248 -> [w254 _]
      frame False {
        n211 = property class="Ctl"(reference=w255, error in=w254, "DisabledEnum"=T3."Enabled" ("Disabled")) -> (error out=w253:errorcluster)  [unwired: 1 out]
        n212 = control-ref of="This VI"() -> (w257:refnum<vi>)
        n213 = property class="VI"(reference=w257, error in=w253, "Front Panel.IsFrontmost"=TRUE ("Front Panel Window:Is Frontmost")) -> (error out=w256:errorcluster)  [unwired: 1 out]
        n214 = call "_PC_Err write_error_message.vi"("show msg( T )"=TRUE, "error in"=w256) -> ()  [unwired: 9 in, 1 out]
      }
      frame True {
      }
    }
  }
  n215 = control-ref of="MS.Pause"() -> (w7:refnum<vi>)
  n216 = control-ref of="warning sign"() -> (w8:refnum<vi>)
  n217 = while {
    tunnel: w1 -> [w337]
    stop <- w338 stop-if-true
    # "Guide Command"
    n218 = event shown="[6] \"Group Name Selection\": Value Change" {
      selector: _ -> [_ _ _ _ _ _ _ _ _ _]
      dyn-events: _ -> [_ _ _ _ _ _ _ _ _ _]
      timeout: _ -> [_ _ _ _ _ _ _ _ _ _]
      tunnel: [_ _ _ _ _ _ _ _ _ w396] -> w338
      tunnel: w337 -> [w339 _ _ _ _ w378 w381 w384 _ w395]
      tunnel: [w339 w340 w345 w362 _ w377 w380 w383 w385 w395] -> w335
      event Timeout {
        n219 = event-data() -> ()  [unwired: 1 in, 1 out]
      }
      event "massSpec": Shortcut Menu Selection (App) {
        n220 = event-data() -> ("CtlRef"=w342:refnum<vi>, "ItemTag"=w341:string)  [unwired: 1 in]
        n221 = case shown="\"APP_SC_PLOT_LEGEND\"" w341 {
          tunnel: w342 -> [_ w344]
          tunnel: [_ w343] -> w340
          frame "False", Default {
          }
          frame "APP_SC_PLOT_LEGEND" {
            n222 = invoke class="XYGraph (strict)" method="FitControlToPane"(reference=w344) -> (error out=w343:errorcluster)  [unwired: 2 in, 2 out]
          }
        }
      }
      event "massSpec": Plot Attribute Change {
        n223 = event-data() -> ("PlotIdx"=w350:i32, "NewAttrib.Color"=w349:u32, "NewAttrib.LineWidth"=w348:u8)  [unwired: 1 in]
        n224 = call "FGV_PlotStyle.vi"("Function"=enum16{"Set", "Get"}."Get") -> ("error out"=w346:errorcluster, "Output Cluster"=w354:T13)  [unwired: 9 in]
        n225 = Unbundle By Name(w354) -> ("LineColorArray"=w358:u32[], "LineWidthArray"=w357:u8[])
        n226 = Replace Array Subset(array=w358, new element=w349, index=w350) -> (w356:u32[])
        n227 = Replace Array Subset(array=w357, new element=w348, index=w350) -> (w355:u8[])
        n228 = Bundle By Name(cluster=w354, "LineColorArray"=w356, "LineWidthArray"=w355) -> (w353:T13)
        n229 = call "FGV_PlotStyle.vi"("Function"=enum16{"Set", "Get"}."Set", "Input Cluster"=w353) -> ("error out"=w347:errorcluster)  [unwired: 8 in, 1 out]
        n230 = Merge Errors(w347, w346) -> (w345:errorcluster)
      }
      event "TIC_wfm", "Ionisation": Shortcut Menu Selection (User) {
        n231 = event-data() -> ("ItemTag"=w364:string)  [unwired: 1 in, 1 out]
        n232 = control-ref of="Ionisation"() -> (w359:refnum<vi>)
        n233 = case shown="\"Ionisation\"" w364 {
          tunnel: [FALSE TRUE] -> w365
          tunnel: [TRUE FALSE] -> w366
          frame "Ionisation" {
          }
          frame "TIC", Default {
          }
        }
        n234 = control-ref of="TIC_wfm"() -> (w360:refnum<vi>)
        n235 = property class="WFGraph (strict)"(reference=w359, "Visible"=w366) -> (error out=w361:errorcluster)  [unwired: 1 in, 1 out]
        n236 = property class="XYGraph (strict)"(reference=w360, "Visible"=w365) -> (error out=w363:errorcluster)  [unwired: 1 in, 1 out]
        n237 = Merge Errors(w363, w361) -> (w362:errorcluster)
      }
      event "Ionisation", "TIC_wfm": Shortcut Menu Activation? {
        w372 = string[] ["TIC", "Ionisation"] ("item names")
        n238 = event-data() -> ("MenuRef"=w373:refnum<k9>)  [unwired: 1 in]
        n239 = Delete Menu Items(9:w373) -> (0:w375:errorcluster, 3:w374:refnum<k9>)  [unwired: 3 in]
        n240 = Insert Menu Items(6:w375, 7:w372, 8:w372, 9:w374) -> ()  [unwired: 2 in, 3 out]
        n241 = event-data("Discard?"=FALSE) -> ()  [unwired: 1 in, 1 out]
      }
      event "Add GroupName": Value Change {
        n242 = event-data() -> ()  [unwired: 1 in, 1 out]
        n243 = call "_PC_Pub_FM ctrlInstrRefNum.vi"("function"=_PC_Pub_FM_ctrlFileRefnumEnum."addNewFileName", "error in (no error)"=w378) -> ("error out"=w377:errorcluster)  [unwired: 9 in]
      }
      event "Group Name Selection": Value Change {
        n244 = event-data() -> ()  [unwired: 1 in, 1 out]
        n245 = call "_PC_Pub_FM ctrlInstrRefNum.vi"("function"=_PC_Pub_FM_ctrlFileRefnumEnum."updFileName", "error in (no error)"=w381) -> ("error out"=w380:errorcluster)  [unwired: 9 in]
      }
      event "Working Folder": Value Change {
        n246 = event-data() -> ()  [unwired: 1 in, 1 out]
        n247 = call "_PC_Pub_FM ctrlInstrRefNum.vi"("function"=_PC_Pub_FM_ctrlFileRefnumEnum."updWorkFolder", "error in (no error)"=w384) -> ("error out"=w383:errorcluster)  [unwired: 9 in]
      }
      event Menu Selection (User) {
        n248 = event-data() -> ("ItemTag"=w386:string)  [unwired: 1 in]
        n249 = case shown="\"AutoSave\"" w386 {
          tunnel: [_ w387] -> w385
          frame Default {
          }
          frame "AutoSave" {
            n250 = call "_PC_Pub ctrlRegistry.vi"("type"=enum16{"None", "Write", "Read"}."Read", "function"=RegistyFunc."FileAutoSave") -> ("error out"=w394:errorcluster, "Boolean output"=w392:bool)  [unwired: 6 in, 2 out]
            n251 = Not(x=w392) -> (.not. x?=w393:bool)
            n252 = call "_PC_Pub ctrlRegistry.vi"("type"=enum16{"None", "Write", "Read"}."Write", "function"=RegistyFunc."FileAutoSave", "error in (no error)"=w394, "write value"=w393) -> ("error out"=w387:errorcluster)  [unwired: 4 in, 3 out]
          }
        }
      }
      event "Stop": Value Change {
        n253 = event-data() -> ("NewVal"=w396:bool)  [unwired: 1 in]
      }
    }
    n254 = call "_PC_Err write_error_message.vi"("show msg( T )"=TRUE, "error in"=w335) -> ()  [unwired: 9 in, 1 out]
  }
  n255 = control-ref of="MS.Laser"() -> (w11:refnum<vi>)
  n256 = control-ref of="Stop"() -> (w10:refnum<vi>)
  n257 = disable-structure shown="Enabled" {
    disable-tunnel: w1 -> [w400 _]
    frame Enabled {
      w401 = FALSE
      # "Permanent"
      n258 = control-ref of="Toolbar Splitter"() -> (w419:refnum<vi>)
      n259 = control-ref of="Monitor Splitter"() -> (w415:refnum<vi>)
      n260 = control-ref of="Smooth.edit"() -> (w411:refnum<vi>)
      n261 = control-ref of="eng_mode_str"() -> (w410:refnum<vi>)
      n262 = control-ref of="Instrument_param_table"() -> (w412:refnum<vi>)
      n263 = property class="Tbl (strict)"(reference=w412, error in=w400, "DisabledEnum"=T3."Disabled" ("Disabled")) -> (reference out=w405:refnum<vi>)  [unwired: 1 out]
      n264 = property class="Splitter"(reference=w419, error in=w400, "Position"=108 ("Splitter Position")) -> (reference out=w417:refnum<vi>)  [unwired: 1 out]
      n265 = property class="Splitter"(reference=w415, error in=w400, "Position"=260 ("Splitter Position")) -> (reference out=w416:refnum<vi>)  [unwired: 1 out]
      n266 = property class="Str"(reference=w410, error in=w400, "Text.FontBold"=TRUE ("Text.Font:Bold"), "Text.FontColor"=u32 16711680, "Value"="Eng. Mode", "Visible"=w401) -> (reference out=w402:refnum<vi>)  [unwired: 1 out]
      n267 = control-ref of="Config Tab"() -> (w414:refnum<vi>)
      n268 = property class="Bool"(reference=w411, error in=w400, "Visible"=w401) -> (reference out=w404:refnum<vi>)  [unwired: 1 out]
      n269 = control-ref of="D999_list"() -> (w399:refnum<vi>)
      n270 = control-ref of="sys_value_list"() -> (w398:refnum<vi>)
      n271 = New Data Value Reference(data value=w401, error in=w400) -> (data value reference=w403:refnum<data-value>)  [unwired: 1 out]
      n272 = while {
        shift-right: [w426] -> _
        shift-left: 0 -> [w427]
        tunnel: w403 -> [w425]
        tunnel: w402 -> [w424]
        tunnel: w404 -> [w423]
        tunnel: w405 -> [w422]
        tunnel: 500 -> [w421]
        stop <- w428 stop-if-true
        # "Operating status"
        n273 = event shown="[0] Timeout" {
          selector: _ -> [_ _ _ _ _ _ _]
          dyn-events: _ -> [_ _ _ _ _ _ _]
          timeout: w421 -> [_ _ _ _ _ _ _]
          tunnel: [_ _ _ _ _ w515 _] -> w428
          tunnel: w427 -> [_ _ _ w482 w491 _ _]
          tunnel: [_ _ _ w482 w490 _ _] -> w426
          tunnel: w425 -> [_ _ _ _ w489 _ _]
          tunnel: w424 -> [_ _ _ _ w488 _ _]
          tunnel: w423 -> [_ _ _ _ w487 _ _]
          tunnel: w422 -> [_ _ _ _ w486 _ _]
          event Timeout {
            n274 = event-data() -> ()  [unwired: 1 in, 3 out]
          }
          event "Instrument_param_table": Value Change {
            n275 = event-data() -> ("CtlRef"=w432:refnum<vi>, "NewVal"=w431:string[][])  [unwired: 1 in]
            n276 = for {
              tunnel: w431 -> [w460] mode=indexing
              shift-right: [w461] -> w435
              shift-left: i32[] [] -> [w462]
              tunnel: [w449] -> w437 mode=indexing
              tunnel: "\\s" -> [w452]
              i -> [w463]
              n277 = Index Array(array=w460) -> (element #1=w457:string, element #2=w456:string)  [unwired: 2 in]
              n278 = Match Pattern(string=w457, regular expression=w452) -> (match substring=w459:string)  [unwired: 1 in, 3 out]
              n279 = Empty String/Path?(string/path=w457) -> (empty?=w454:bool)
              n280 = Empty String/Path?(string/path=w456) -> (empty?=w453:bool)
              n281 = Empty String/Path?(string/path=w459) -> (empty?=w458:bool)
              n282 = Build Array(w454, w453) -> (w455:bool[])
              n283 = Not(x=w458) -> (.not. x?=w449:bool)
              n284 = And Array Elements(Boolean array=w455) -> (logical AND=w450:bool)
              n285 = Or(x=w450, y=w449) -> (x .or. y?=w451:bool)
              n286 = case shown="True" w451 {
                tunnel: w463 -> [_ w466]
                tunnel: w462 -> [w464 w467]
                tunnel: [w464 w465] -> w461
                frame False {
                }
                frame True {
                  n287 = Build Array (concatenate)(w467, w466) -> (w465:i32[])
                }
              }
            }
            n288 = Reverse 1D Array(array=w435) -> (reversed array=w436:i32[])
            n289 = Or Array Elements(Boolean array=w437) -> (logical OR=w438:bool)
            n290 = case shown="True" w438 {
              frame False {
              }
              frame True {
                n291 = One Button Dialog(message="Do not accept space characters") -> ()  [unwired: 1 in, 1 out]
              }
            }
            n292 = for {
              tunnel: w436 -> [w447] mode=indexing
              shift-right: [w446] -> w429
              shift-left: w431 -> [w448]
              n293 = Delete From Array(array=w448, index (row)=w447) -> (array with subset deleted=w446:string[][])  [unwired: 2 in, 1 out]
            }
            n294 = property class="Tbl (strict)"(reference=w432, "Value"=w429) -> (error out=w430:errorcluster)  [unwired: 1 in, 1 out]
            n295 = case shown="No Error" w430 {
              tunnel: w429 -> [w440 _]
              frame No Error {
                n296 = Two Button Dialog(message="Access new parameter?") -> (T button?=w441:bool)  [unwired: 2 in]
                n297 = case shown="True" w441 {
                  tunnel: w440 -> [_ w444]
                  tunnel: "System" ("add tag name") -> [_ w443]
                  frame False {
                  }
                  frame True {
                    n298 = call "DataXML saveXMLProcess.vi"("addTagName"=w443, "newData"=w444) -> ()  [unwired: 9 in, 1 out]
                  }
                }
              }
              frame Error {
              }
            }
          }
          event "Instrument_param_table": Mouse Down? {
            n299 = event-data() -> ("CtlRef"=w481:refnum<vi>, "Coords"=w480:T14)  [unwired: 1 in]
            n300 = invoke class="Tbl (strict)" method="Point To Row Column"(reference=w481, "Point"=w480) -> (reference out=w470:refnum<vi>, error out=w469:errorcluster, "CellPosition"=w471:T15)  [unwired: 4 in, 3 out]
            n301 = property class="Tbl (strict)"(reference=w470, error in=w469) -> ("Value"=w478:string[][])  [unwired: 2 out]
            n302 = Array Size(array=w478) -> (size(s)=w477:i32[])
            n303 = Index Array(array=w477, index=0) -> (element=w474:i32)
            n304 = Unbundle By Name(w471) -> ("Row"=w475:i32, "Column"=w479:i32)
            n305 = Equal To 0?(x=w479) -> (x = 0?=w472:bool)
            n306 = Greater Or Equal?(x=w475, y=w474) -> (x >= y?=w473:bool)
            n307 = Or(x=w473, y=w472) -> (x .or. y?=w468:bool)
            n308 = event-data("Discard?"=w468) -> ()  [unwired: 1 in, 1 out]
          }
          event Mouse Move {
            n309 = event-data() -> ()  [unwired: 1 in, 1 out]
            n310 = call "_PC_Pub ctrlRegistry.vi"("type"=enum16{"None", "Write", "Read"}."Write", "function"=RegistyFunc."ExeStatu", "write value"=u32 1) -> ()  [unwired: 5 in, 4 out]
          }
          event Key Down {
            n311 = event-data() -> ("Char"=w492:i16)  [unwired: 1 in]
            n312 = case shown="121" w492 {
              tunnel: w491 -> [_ w501]
              tunnel: [_ w497] -> w490
              tunnel: w489 -> [_ w496]
              tunnel: w488 -> [_ w495]
              tunnel: w487 -> [_ w494]
              tunnel: w486 -> [_ w493]
              frame 0, Default {
              }
              frame 121 {
                n313 = Increment(x=w501) -> (x+1=w498:i32)
                n314 = Greater?(x=w498, y=4) -> (0:w499:bool)
                n315 = case shown="True" w499 {
                  tunnel: w498 -> [w502 _]
                  tunnel: [w502 _] -> w497
                  tunnel: w496 -> [_ w506]
                  tunnel: w495 -> [_ w505]
                  tunnel: w494 -> [_ w504]
                  tunnel: w493 -> [_ w503]
                  frame False {
                  }
                  frame True {
                    n316 = in-place {
                      in-place-border: w505 -> [w513]
                      in-place-border: w504 -> [w512]
                      in-place-border: w503 -> [w511]
                      n317 = in-place-dvr #2(w506) -> (w514:bool)  [unwired: 1 out]
                      n318 = Not(x=w514) -> (.not. x?=w510:bool)
                      n319 = Select(t=T3."Enabled" ("Disabled"), s=w510, f=T3."Disabled") -> (s? t:f=w507:T3)
                      n320 = property class="Str"(reference=w513, "Visible"=w510) -> ()  [unwired: 1 in, 2 out]
                      n321 = property class="Bool"(reference=w512, "Visible"=w510) -> ()  [unwired: 1 in, 2 out]
                      n322 = property class="Tbl (strict)"(reference=w511, "DisabledEnum"=w507) -> ()  [unwired: 1 in, 2 out]
                      n323 = in-place-dvr #2(w510) -> ()  [unwired: 2 out]
                    }
                  }
                }
              }
            }
          }
          event "Stop": Value Change {
            n324 = event-data() -> ("NewVal"=w515:bool)  [unwired: 1 in]
          }
          event "massSpec": Mouse Down? {
            n325 = event-data() -> ("CtlRef"=w517:refnum<vi>, "Mods.Double Click"=w518:bool)  [unwired: 1 in]
            n326 = case shown="True" w518 {
              tunnel: w517 -> [_ w538]
              tunnel: [_ TRUE] -> w516
              frame False {
              }
              frame True {
                n327 = property class="XYGraph (strict)"(reference=w538, "ActPaletteTool"=5 ("Palette:Active Tool")) -> (reference out=w536:refnum<vi>, error out=w535:errorcluster)  [unwired: 1 in]
                n328 = property class="XYGraph (strict)"(reference=w536, error in=w535, "ActXScl"=1 ("Active X Scale")) -> (reference out=w519:refnum<vi>, error out=w533:errorcluster)
                n329 = property class="XYGraph (strict)"(reference=w519, error in=w533) -> (reference out=w520:refnum<vi>, error out=w521:errorcluster, "Plot.Plot Name"=w532:string)
                n330 = Spreadsheet String To Array(delimiter (Tab)=",", format string="%.3f", spreadsheet string=w532, array type (2D Dbl)=dbl[] []) -> (array=w528:dbl[])
                n331 = Index Array(array=w528) -> (element #1=w527:dbl, element #2=w526:dbl)  [unwired: 2 in]
                n332 = property class="XYGraph (strict)"(reference=w520, error in=w521, "XScale.Maximum"=w527, "XScale.Minimum"=w526) -> (reference out=w523:refnum<vi>, error out=w524:errorcluster)
                n333 = property class="XYGraph (strict)"(reference=w523, error in=w524, "ActXScl"=0 ("Active X Scale")) -> ()  [unwired: 2 out]
              }
            }
            n334 = event-data("Discard?"=w516) -> ()  [unwired: 1 in, 1 out]
          }
        }
      }
      n335 = while {
        tunnel: w414 -> [w543]
        tunnel: w417 -> [w542]
        tunnel: w416 -> [_]
        tunnel: w399 -> [w540]
        tunnel: w398 -> [w539]
        stop <- w541 stop-if-true
        # "SubPanel Splitter Events"
        n336 = event shown="[1] \"Toolbar Splitter\": Mouse Down" {
          selector: _ -> [_ _ _ _ _]
          dyn-events: _ -> [_ _ _ _ _]
          timeout: _ -> [_ _ _ _ _]
          tunnel: w543 -> [_ w547 w550 w551 _]
          tunnel: w542 -> [_ w546 _ _ _]
          tunnel: [_ _ _ _ w553] -> w541
          tunnel: w540 -> [_ w545 w549 _ _]
          tunnel: w539 -> [_ w544 w548 _ _]
          event Timeout {
            n337 = event-data() -> ()  [unwired: 1 in, 1 out]
          }
          event Mouse Down {
            n338 = event-data() -> ()  [unwired: 1 in, 1 out]
            n339 = call "_PC_Pub_Splitter_ToolbarWindow.vi"("sys_value_list"=w544, "d999_list"=w545, "Config Tab"=w547, "SplitterRef"=w546) -> ()  [unwired: 1 in]
          }
          event Panel Resize {
            n340 = event-data() -> ()  [unwired: 1 in, 1 out]
            n341 = call "_PC_Pub_Splitter_ResizeWindow.vi"("sys_value_list"=w548, "d999_list"=w549, "Config Tab"=w550) -> ()  [unwired: 1 in]
          }
          event Mouse Down {
            n342 = event-data() -> ("SplitterRef"=w552:refnum<vi>)  [unwired: 1 in]
            n343 = call "_PC_Pub_Splitter_ConfigWindow.vi"("Config Tab"=w551, "SplitterRef"=w552) -> ()  [unwired: 1 in]
          }
          event "Stop": Value Change {
            n344 = event-data() -> ("NewVal"=w553:bool)  [unwired: 1 in]
          }
        }
      }
    }
    frame Disabled {
    }
  }
  n345 = control-ref of="Version :"() -> (w28:refnum<vi>)
  n346 = call "interfaceLoop idleStateCheck.vi"("laserRefnum"=w11, "error in (no error)"=w1, "connectStateRefnum"=w9, "Stop"=w10) -> ()  [unwired: 7 in, 1 out]
  n347 = call "_PC_MS_SubVI writeToTDMS.vi"("MS.Pause"=w7, "warning sign"=w8, "error in (no error)"=w1, "Stop"=w10) -> ()  [unwired: 7 in, 1 out]
  n348 = call "interfaceLoop systemRecord.vi"("Version :"=w28, "error in (no error)"=w1, "connectStateRefnum"=w9, "Stop"=w10) -> ()  [unwired: 7 in, 1 out]
  n349 = call "interfaceLoop firmwareStateCheck.vi"("error in (no error)"=w1, "connectStateRefnum"=w9, "Stop"=w10) -> ()  [unwired: 8 in, 1 out]
  n350 = call "interfaceLoop tabStateCheck.vi"("error in (no error)"=w1, "connectStateRefnum"=w9, "Stop"=w10) -> ()  [unwired: 8 in, 1 out]
